vi "Create from CSV Row.vi"(8 "error in (no error)":errorcluster, 11 "CSV Row":string) -> (0 "error out":errorcluster, 3 "Credit Record out":refnum<class "Credit Transaction.lvclass">)   [LabVIEW 2018, in "Credit Transaction.lvclass"]
uses:
  Credit Transaction.lvclass
  C:/GitRepos/Filthy-Lucre-Budgetizer/source/support/classes/Transaction/Transaction.lvclass
  <vilib>/Utility/miscctls.llb/LVDateTimeRec.ctl
  Transaction/Transaction.lvclass
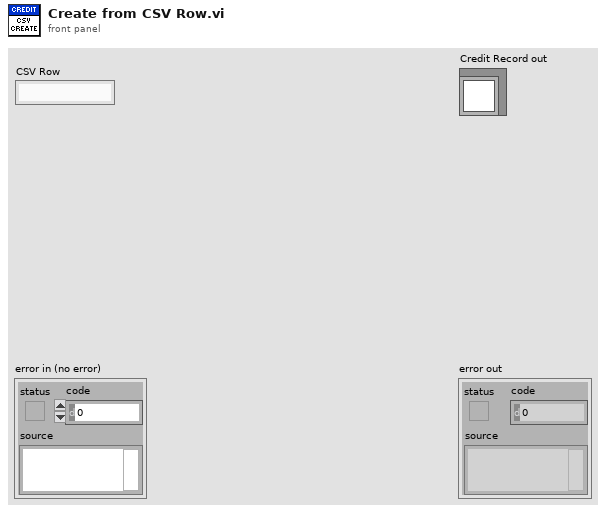
[diagram p1: front panel]
types:
  T1 = typedef "LVDateTimeRec.ctl" = cluster{"fractional second":dbl, "second":i32, "minute":i32, "hour":i32, "day of month":i32, "month":i32, "year":i32, "day of week":i32, "day of year":i32, "DST":i32}
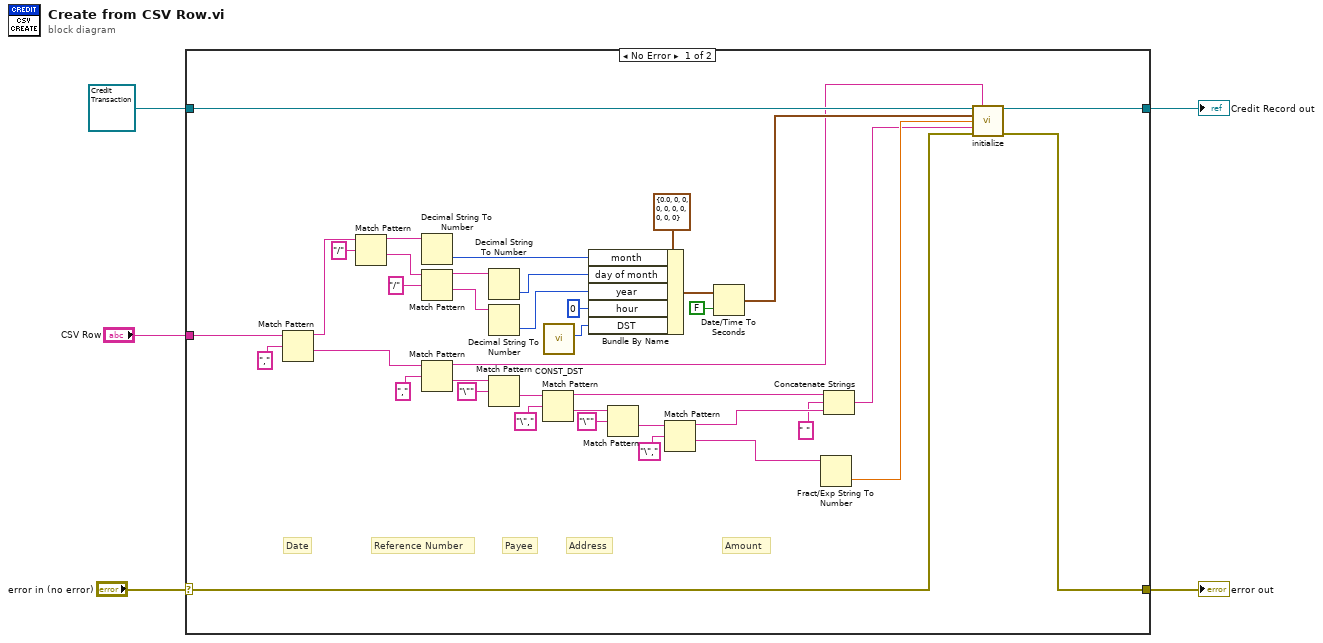
[diagram p0: block diagram]
diagram:
  n1 = case shown="No Error" "error in (no error)" {
    selector: "error in (no error)" -> [w19 w46]
    tunnel: [w43 w46] -> w4
    tunnel: [w7 w45] -> w2
    tunnel: refnum<class "Credit Transaction.lvclass"> refnum ("Credit Record in") -> [w44 w45]
    tunnel: "CSV Row" -> [w18 _]
    frame No Error {
      # "Amount"
      # "Reference Number"
      # "Payee"
      # "Address"
      # "Date"
      n2 = Match Pattern(string=w18, regular expression=",") -> (before substring=w21:string, after substring=w13:string)  [unwired: 3 out]
      n3 = Match Pattern(string=w21, regular expression="/") -> (before substring=w30:string, after substring=w28:string)  [unwired: 3 out]
      n4 = Decimal String To Number(string=w30) -> (number=w27:i32)  [unwired: 2 in, 1 out]
      n5 = Match Pattern(string=w28, regular expression="/") -> (before substring=w26:string, after substring=w24:string)  [unwired: 3 out]
      n6 = Match Pattern(string=w13, regular expression=",") -> (before substring=w6:string, after substring=w38:string)  [unwired: 3 out]
      n7 = Decimal String To Number(string=w26) -> (number=w25:i32)  [unwired: 2 in, 1 out]
      n8 = Decimal String To Number(string=w24) -> (number=w23:i32)  [unwired: 2 in, 1 out]
      n9 = Match Pattern(string=w38, regular expression="\"") -> (after substring=w40:string)  [unwired: 4 out]
      n10 = Match Pattern(string=w40, regular expression="\",") -> (before substring=w16:string, after substring=w34:string)  [unwired: 3 out]
      n11 = call "CONST_DST.vi"() -> ("DST"=w8:i32)  [unwired: 11 in]
      n12 = Bundle By Name(cluster=T1 {"fractional second"=0.0, "second"=0, "minute"=0, "hour"=0, "day of month"=0, "month"=0, "year"=0, "day of week"=0, "day of year"=0, "DST"=0} ("date time rec"), "month"=w27, "day of month"=w25, "year"=w23, "hour"=0, "DST"=w8) -> (w33:T1)
      n13 = Match Pattern(string=w34, regular expression="\"") -> (after substring=w36:string)  [unwired: 4 out]
      n14 = Match Pattern(string=w36, regular expression="\",") -> (before substring=w15:string, after substring=w12:string)  [unwired: 3 out]
      n15 = Date/Time To Seconds(1:FALSE ("is UTC (F)"), 2:w33) -> (0:w17:timestamp)
      n16 = Fract/Exp String To Number(string=w12) -> (number=w11:dbl)  [unwired: 3 in, 1 out]
      n17 = Concatenate Strings(w16, " ", w15) -> (w10:string)
      n18 = call "initialize.vi"("Transaction in"=w44, "Reference"=w6, "Date"=w17, "Amount"=w11, "Description"=w10, "error in (no error)"=w19) -> ("Transaction out"=w7:refnum<class "Credit Transaction.lvclass">, "error out"=w43:errorcluster)  [unwired: 8 in]
    }
    frame Error {
    }
  }
  "error out" <- w4
  "Credit Record out" <- w2
